vi "API Color Sensor Get Color.vi"(9 "Blue Input":i32, 10 "Green Input":i32, 11 "Red Input":i32) -> (0 "ColorSendor Return Value":bool, 1 "Blue Output":i32, 2 "Green Output":i32, 3 "Red Output":i32)   [LabVIEW 2011, in "API ColorSensor.lvlib"]
uses:
  API ColorSensor.lvlib
  ColorSensor.dll
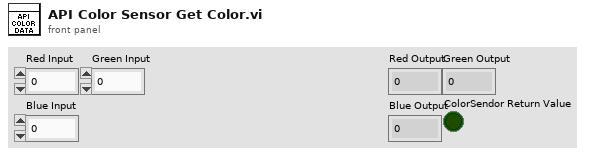
[diagram p1: front panel]
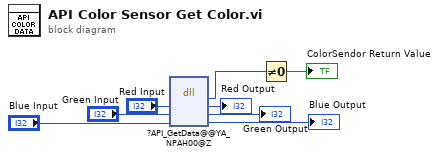
[diagram p0: block diagram]
diagram:
  n1 = dll-call lib="PTH1pabs CUsers\nAdministratorDesktop可重构机电平台项目DemoLabView基础APIColorSensor.dll" fn="?API_GetData@@YA_NPAH00@Z"("Red"="Red Input", "Green"="Green Input", "Blue"="Blue Input") -> ("返回类型"=w2:i32, "Red"=→"Red Output":i32, "Green"=→"Green Output":i32, "Blue"=→"Blue Output":i32)  [unwired: 3 in, 2 out]
  n2 = Not Equal To 0?(x=w2) -> (x != 0?=→"ColorSendor Return Value":bool)
